vi "SPI Communication.vi"() -> ()   [LabVIEW 2023]
doc: "Overview\nDemonstrates how to use the NI-Digital Pattern Driver API to create and configure an instrument session and to burst a pattern on the digital pattern instrument using a start trigger."
uses:
  <instrlib>/niDigital/niDigital.llb/niDigital Pin State.ctl
  <instrlib>/niDigital/niDigital.llb/niDigital Data Mapping.ctl
  <instrlib>/niDigital/niDigital.llb/niDigital Bit Order.ctl
  <instrlib>/niDigital/niDigital.llb/niDigital Write Static Pin State.ctl
  <instrlib>/niDigital/niDigital.llb/niDigital Selected Function.ctl
  <instrlib>/niDigital/niDigital.llb/niDigital Load Specifications Levels and Timing (Single).vi
  <instrlib>/niDigital/niDigital.llb/niDigital Create Source Waveform (Serial).vi
  <instrlib>/niDigital/niDigital.llb/niDigital Create Capture Waveform (Serial).vi
  <instrlib>/niDigital/niDigital.llb/niDigital Write Source Waveform (Site Unique U32).vi
  <instrlib>/niDigital/niDigital.llb/niDigital Burst Pattern (Pass Fail).vi
  <instrlib>/niDigital/niDigital.llb/niDigital Output Function.ctl
panel:
  out "Command Value hex":u32[](array[numeric]) format="%.0x"
  in  "Write/Read":bool
  out "Command Value":u32[](array[numeric])
  out "Digital Data Out":bool[][](array[boolean])
  out "Burst Passed":bool
  out "DUT up":bool
  in  "LowStop":bool
  out "Read Value":u32[](array[numeric]) format="%.0x"
  in  "Write Value":u8[](array[numeric])=[16] format="%.0x"
  in  "Register Address":u8[](array[numeric])=[16] format="%.0x"
  in  "Digital Pattern Resource":refnum<k15>="HSD_6571_C02_S03" caption="resource name"
  in  "Debugg":bool
  in  "Write":bool
  in  "Read":bool
  out "Sequence Flags":bool[](array[boolean])
  out "Sequence Register":i32[](array[numeric])
  out "DIO State":cluster{"channel list":string, "data":T1}[](array[cluster]) {"data" items=["0"=0, "1"=1, "L"=3, "H"=4, "X"=5, "M"=6, "V"=7, "D"=8, "E"=9, "Not A Pin State"=254, "Pin State Not Acquired"=255]}
  out "error out":errorcluster
  # "!"
  # "In CTRL_REG1 set bit 1 to select 3 wire SPI instead of 4 wire.\nBei default it is 0."
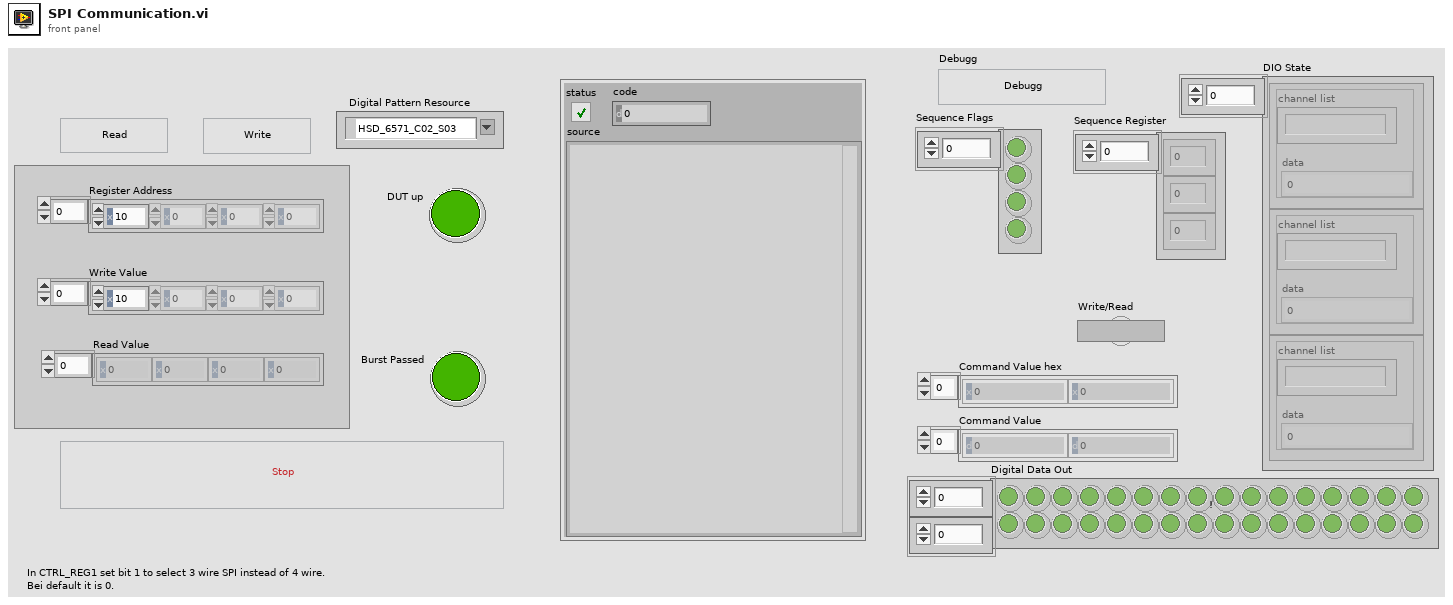
[diagram p1: front panel]
types:
  T1 = typedef "niDigital Pin State.ctl" = u8
  T2 = typedef "niDigital Bit Order.ctl" = i32
  T3 = typedef "niDigital Data Mapping.ctl" = i32
  T4 = typedef "niDigital Output Function.ctl" = i32
  T5 = typedef "niDigital Selected Function.ctl" = i32
  T6 = typedef "niDigital Write Static Pin State.ctl" = u8
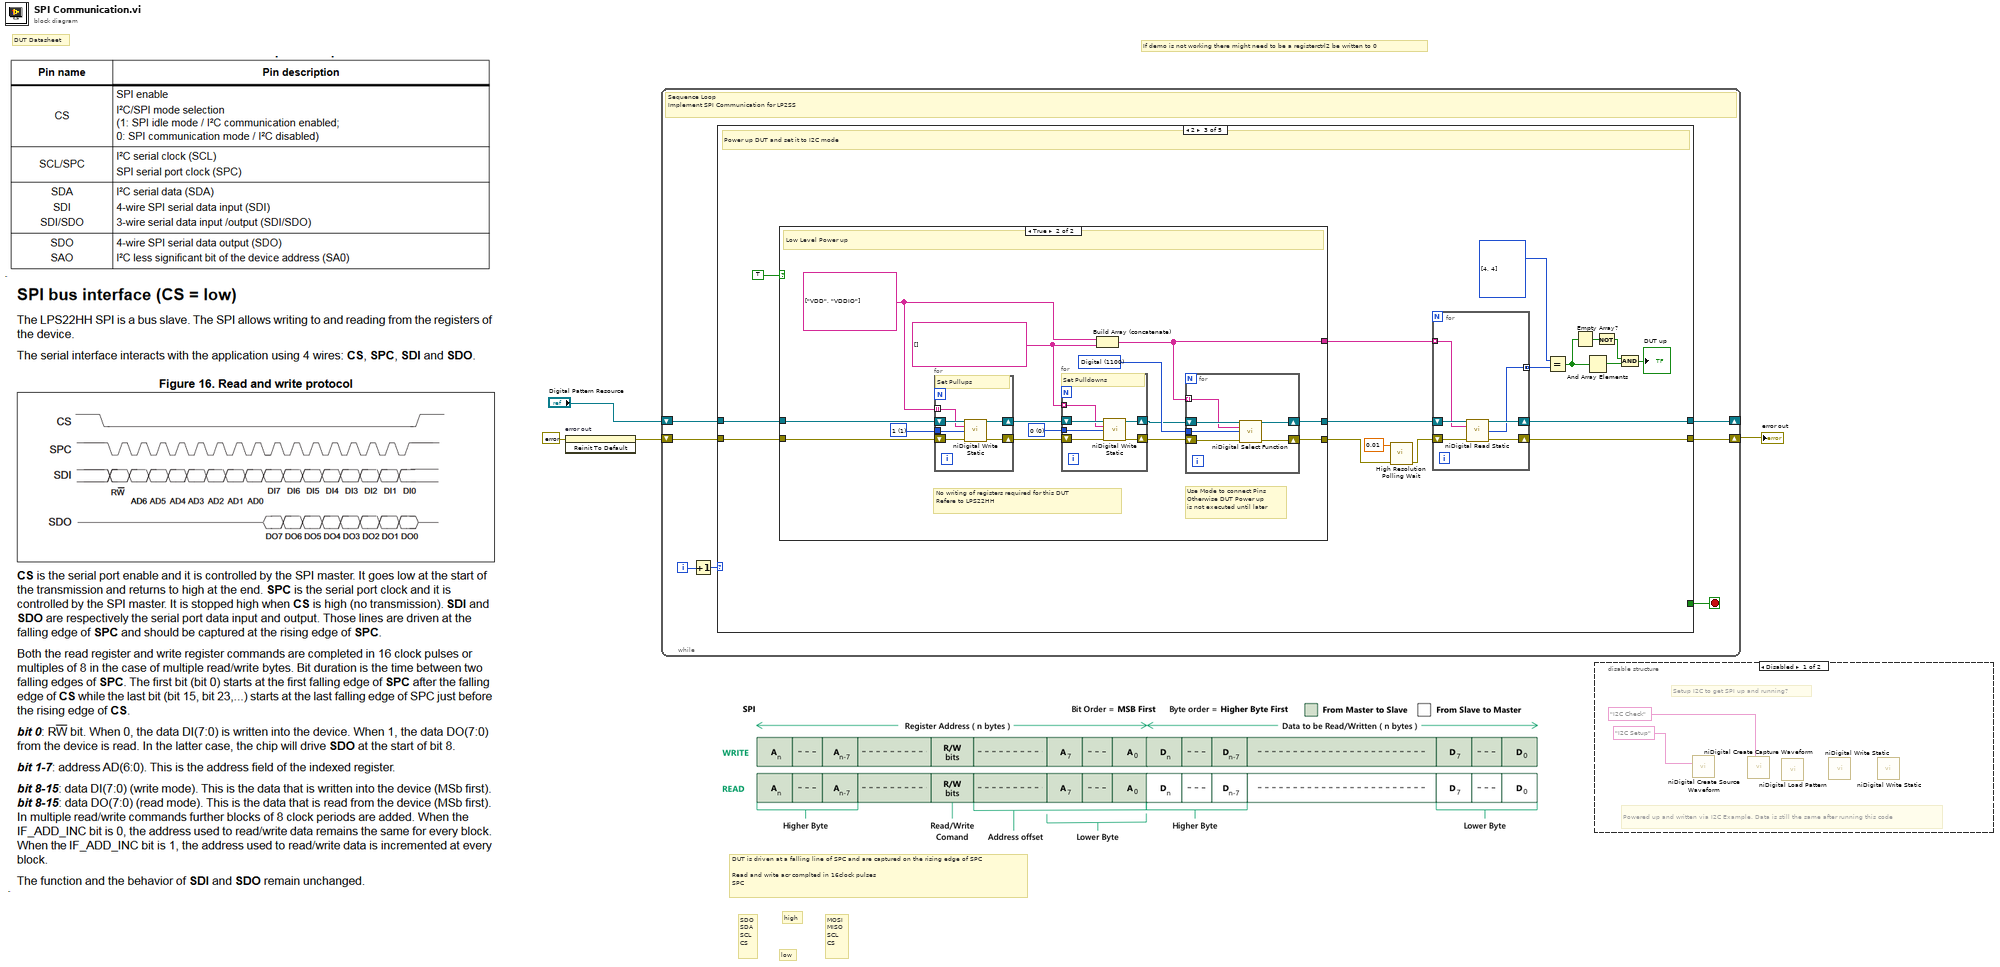
[diagram p0: block diagram]
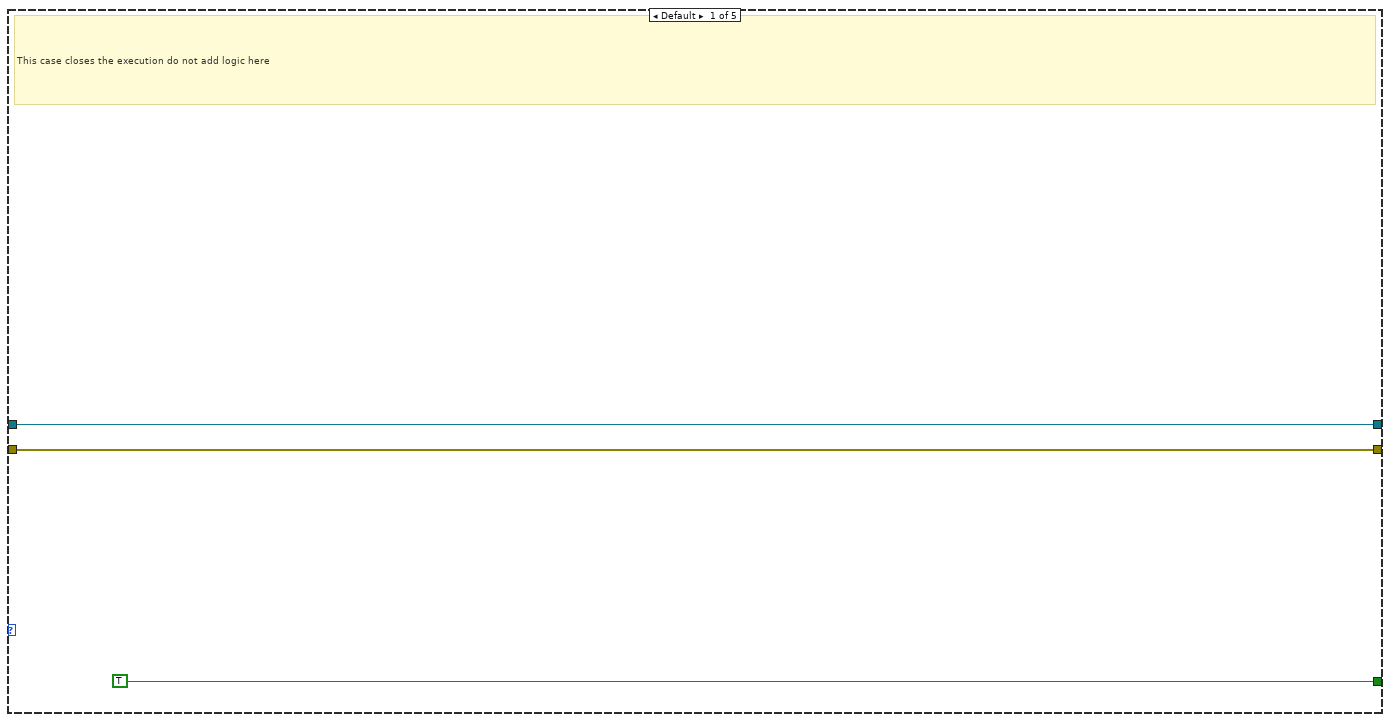
[diagram p3: hidden frame]
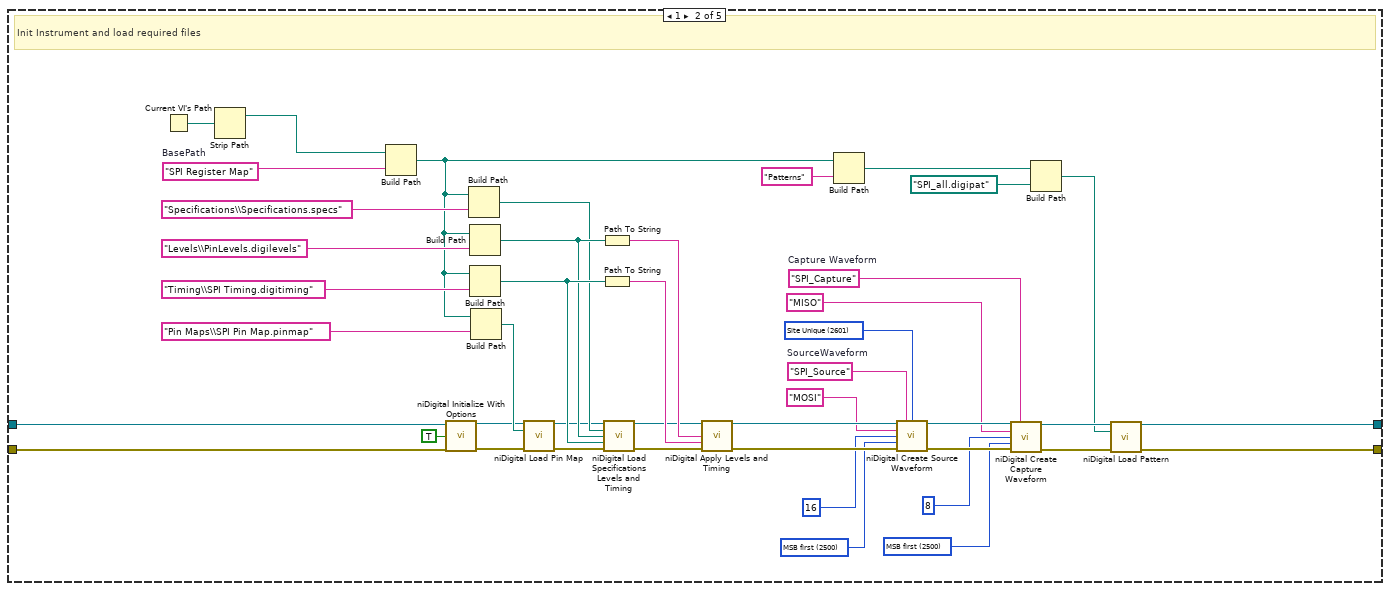
[diagram p4: hidden frame]
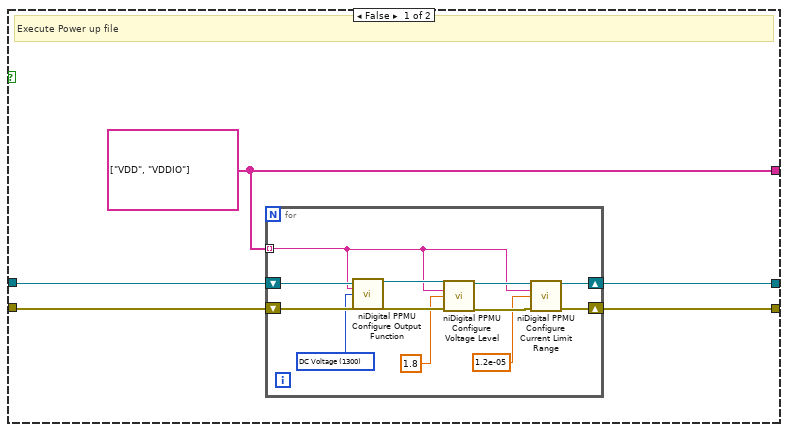
[diagram p5: hidden frame]
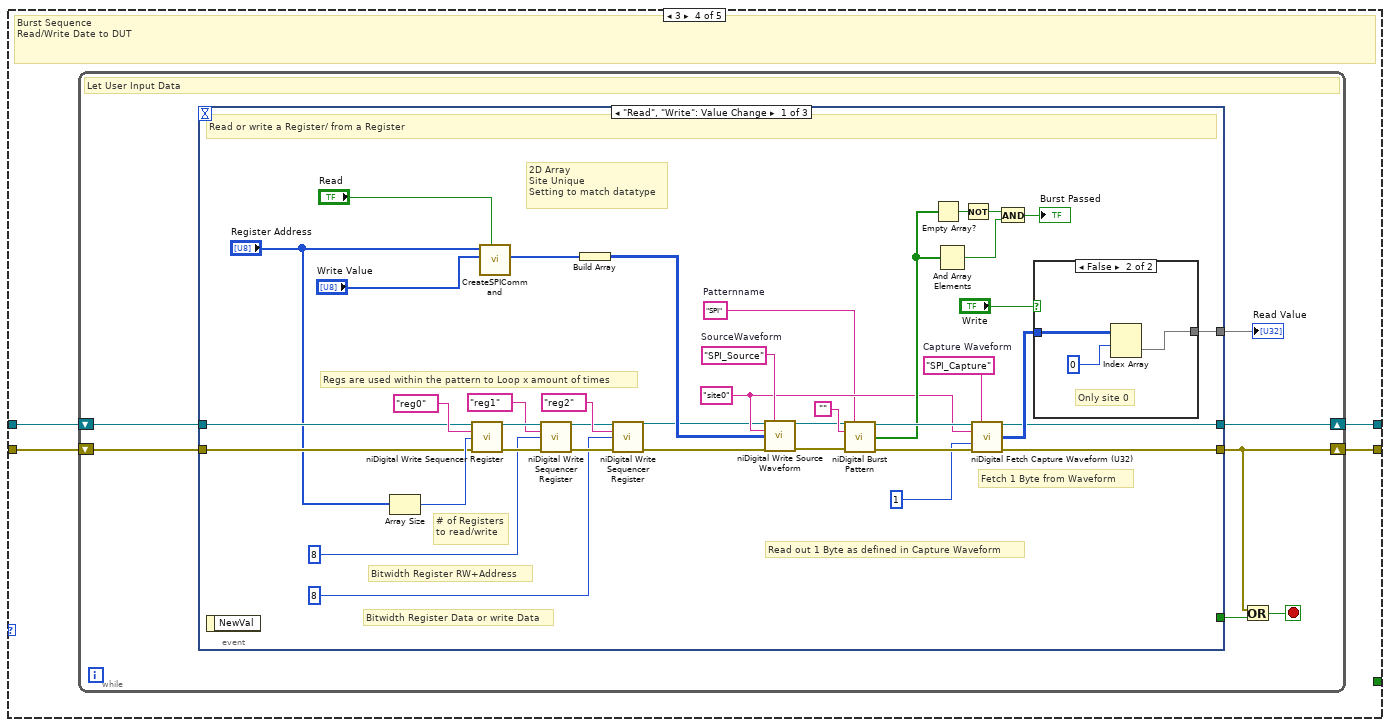
[diagram p6: hidden frame]
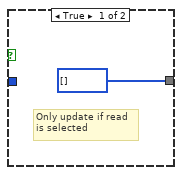
[diagram p7: hidden frame]
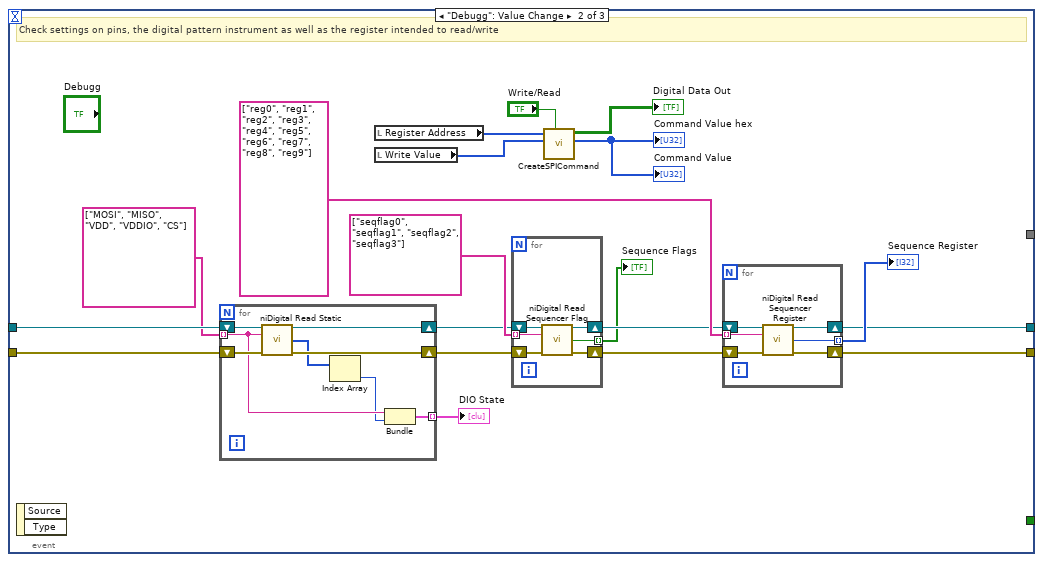
[diagram p8: hidden frame]
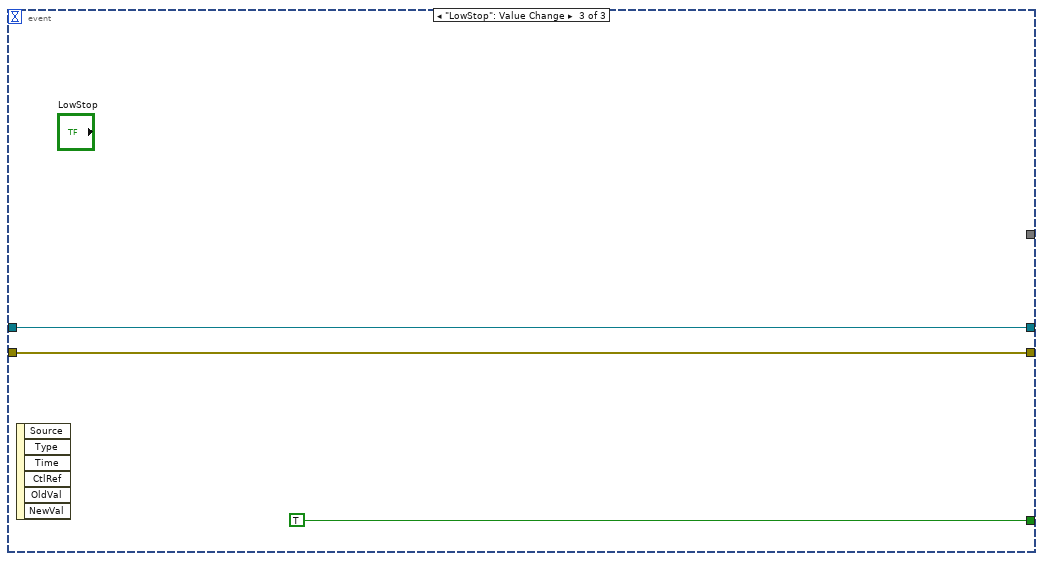
[diagram p9: hidden frame]
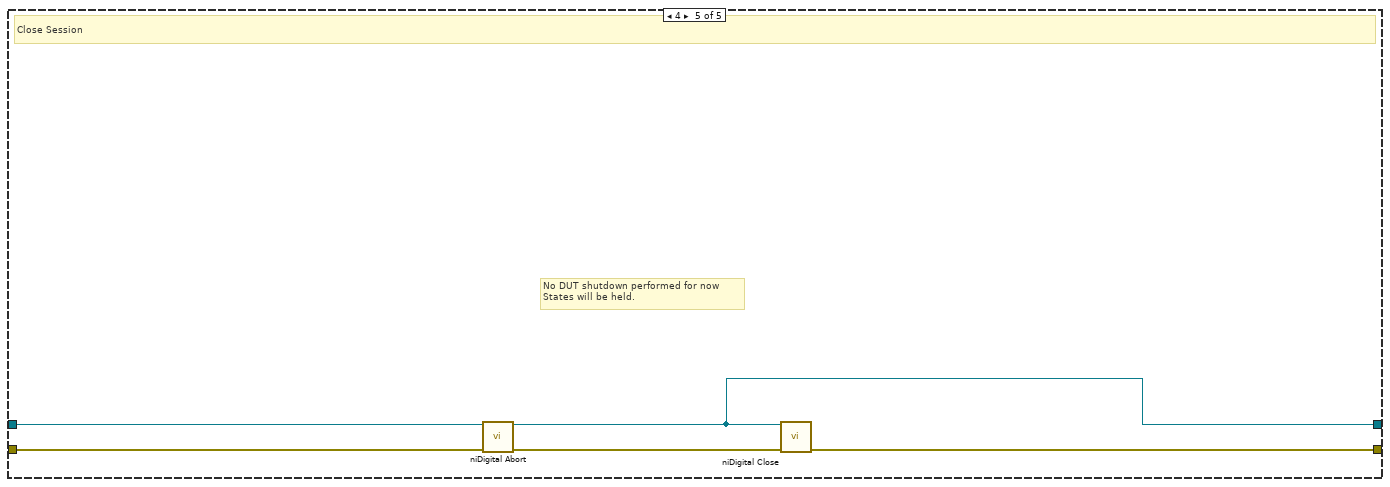
[diagram p10: hidden frame]
diagram:
  # "If demo is not working there might need to be a registerctrl2 be written to 0"
  # "MOSI\nMISO\nSCL\nCS"
  # "high"
  # "low"
  # "SDO\nSDA\nSCL\nCS"
  # "DUT Datasheet"
  # "DUT is driven at a falling line of SPC and are captured on the rising edge of SPC\n\nRead and write acr complted in 16clock pulses\nSPC"
  n1 = invoke on="error out" class="Clust (strict)" method="Reinit To Default"(error in=errorcluster {"status"=FALSE, "code"=0, "source"=""} ("error out")) -> (error out=w3:errorcluster)  [unwired: 2 in, 2 out]
  n2 = while {
    shift-right: [w11] -> w2
    shift-left: w3 -> [w7]
    shift-right: [w6] -> _
    shift-left: "Digital Pattern Resource" -> [w5]
    i -> [w9]
    stop <- w10 stop-if-true
    # "Sequence Loop\nImplement SPI Communication for LP2SS"
    n3 = Increment(x=w9) -> (x+1=w8:i32)
    n4 = case shown="2" w8 {
      tunnel: [w12 w37 w72 w134 w229] -> w6
      tunnel: w5 -> [w12 w28 w74 w133 w227]
      tunnel: w7 -> [w13 w27 w75 w132 w230]
      tunnel: [w13 w38 w73 w131 w231] -> w11
      tunnel: [TRUE _ _ _ _] -> w10
      frame Default {
        # "This case closes the execution do not add logic here"
      }
      frame 1 {
        w16 = T2 2500 items=["MSB first"=2500, "LSB first"=2501] ("bit order")
        w21 = T3 2601 items=["Broadcast"=2600, "Site Unique"=2601] ("data mapping")
        w22 = "SPI_Source"  # SourceWaveform
        w17 = T2 2500 items=["MSB first"=2500, "LSB first"=2501] ("bit order")
        w24 = "SPI_Capture"  # Capture Waveform
        w34 = "SPI Register Map"  # BasePath
        # "Init Instrument and load required files"
        n5 = Current VI's Path() -> (path=w33:path)
        n6 = Strip Path(path=w33) -> (stripped path=w32:path)  [unwired: 1 out]
        n7 = Build Path(base path=w32, name or relative path=w34) -> (appended path=w29:path)
        n8 = call <instrlib>:"niDigital Initialize With Options.vi"("resource name"=w28, "reset (T)"=TRUE, "error in"=w27) -> ("instrument handle"=w50:refnum<k15>, "error out"=w51:errorcluster)  [unwired: 11 in]
        n9 = Build Path(base path=w29, name or relative path="Specifications\\Specifications.specs") -> (appended path=w56:path)
        n10 = Build Path(base path=w29, name or relative path="Levels\\PinLevels.digilevels") -> (appended path=w57:path)
        n11 = Build Path(base path=w29, name or relative path="Timing\\SPI Timing.digitiming") -> (appended path=w58:path)
        n12 = Build Path(base path=w29, name or relative path="Pin Maps\\SPI Pin Map.pinmap") -> (appended path=w55:path)
        n13 = call <instrlib>:"niDigital Load Pin Map.vi"("instrument handle"=w50, "pin map file"=w55, "error in"=w51) -> ("instrument handle out"=w53:refnum<k15>, "error out"=w54:errorcluster)  [unwired: 11 in]
        n14 = Path To String(path=w57) -> (string=w52:string)
        n15 = Path To String(path=w58) -> (string=w49:string)
        n16 = call-poly <instrlib>:"niDigital Load Specifications Levels and Timing.vi"("instrument handle"=w53, "specifications file path"=w56, "levels file path"=w57, "timing file path"=w58, "error in"=w54) -> ("instrument handle out"=w45:refnum<k15>, "error out"=w46:errorcluster)  [unwired: 9 in]
        n17 = call <instrlib>:"niDigital Apply Levels and Timing.vi"("instrument handle"=w45, "levels sheet"=w52, "timing sheet"=w49, "error in"=w46) -> ("instrument handle out"=w48:refnum<k15>, "error out"=w47:errorcluster)  [unwired: 10 in]
        n18 = Build Path(base path=w29, name or relative path="Patterns") -> (appended path=w30:path)
        n19 = call-poly <instrlib>:"niDigital Create Source Waveform.vi"("instrument handle"=w48, "waveform name"=w22, "data mapping"=w21, "pin list"="MOSI", "sample width"=u32 16, "bit order"=w17, "error in"=w47) -> ("instrument handle out"=w25:refnum<k15>, "error out"=w26:errorcluster)  [unwired: 7 in]
        n20 = call-poly <instrlib>:"niDigital Create Capture Waveform.vi"("instrument handle"=w25, "waveform name"=w24, "pin list"="MISO", "sample width"=u32 8, "bit order"=w16, "error in"=w26) -> ("instrument handle out"=w40:refnum<k15>, "error out"=w39:errorcluster)  [unwired: 8 in]
        n21 = Build Path(base path=w30, name or relative path=path "SPI_all.digipat" ("pattern file")) -> (appended path=w35:path)
        n22 = call <instrlib>:"niDigital Load Pattern.vi"("instrument handle"=w40, "pattern file"=w35, "error in"=w39) -> ("instrument handle out"=w37:refnum<k15>, "error out"=w38:errorcluster)  [unwired: 11 in]
      }
      frame 2 {
        w63 = T1[] [4, 4] items=["0"=0, "1"=1, "L"=3, "H"=4, "X"=5, "M"=6, "V"=7, "D"=8, "E"=9, "Not A Pin State"=254, "Pin State Not Acquired"=255]
        # "Power up DUT and set it to I2C mode"
        n23 = case shown="True" TRUE {
          tunnel: w75 -> [w79 w106]
          tunnel: w74 -> [w80 w105]
          tunnel: [w77 w99] -> w65
          tunnel: [w78 w98] -> w61
          tunnel: [w76 w96] -> w64
          frame False {
            w76 = string[] ["VDD", "VDDIO"] ("channel list")
            # "Execute Power up file"
            n24 = for {
              shift-right: [w84] -> w77
              shift-left: w80 -> [w92]
              shift-right: [w85] -> w78
              shift-left: w79 -> [w91]
              tunnel: w76 -> [w82] mode=indexing
              w88 = T4 1300 items=["DC Voltage"=1300, "DC Current"=1301] ("output function")
              n25 = call <instrlib>:"niDigital PPMU Configure Output Function.vi"("instrument handle"=w92, "channel list"=w82, "output function"=w88, "error in"=w91) -> ("instrument handle out"=w90:refnum<k15>, "error out"=w89:errorcluster)  [unwired: 10 in]
              n26 = call <instrlib>:"niDigital PPMU Configure Voltage Level.vi"("instrument handle"=w90, "channel list"=w82, "voltage level (V)"=1.8, "error in"=w89) -> ("instrument handle out"=w83:refnum<k15>, "error out"=w86:errorcluster)  [unwired: 10 in]
              n27 = call <instrlib>:"niDigital PPMU Configure Current Limit Range.vi"("instrument handle"=w83, "channel list"=w82, "current limit range (A)"=1.2e-05 ("current limit (A)"), "error in"=w86) -> ("instrument handle out"=w84:refnum<k15>, "error out"=w85:errorcluster)  [unwired: 10 in]
            }
          }
          frame True {
            w97 = T5 1100 items=["Digital"=1100, "PPMU"=1101, "Off"=1102, "Disconnect"=1103, "RIO"=1104] ("function")
            w100 = string[] [] ("channel list")
            w103 = T6 0 items=["0"=0, "1"=1, "X"=5] ("state")
            w94 = string[] ["VDD", "VDDIO"] ("channel list")
            w104 = T6 1 items=["0"=0, "1"=1, "X"=5] ("state")
            # "Use Mode to connect Pins\nOtherwise DUT Power up \nis not executed until later"
            # "No writing of registers required for this DUT\nRefere to LPS22HH"
            # "Low Level Power up"
            n28 = for {
              tunnel: w104 -> [w122]
              tunnel: w94 -> [w121] mode=indexing
              shift-right: [w120] -> w102
              shift-left: w105 -> [w123]
              shift-right: [w119] -> w101
              shift-left: w106 -> [w124]
              # "Set Pullups"
              n29 = call <instrlib>:"niDigital Write Static.vi"("instrument handle"=w123, "channel list"=w121, "state"=w122, "error in"=w124) -> ("instrument handle out"=w120:refnum<k15>, "error out"=w119:errorcluster)  [unwired: 10 in]
            }
            n30 = for {
              tunnel: w103 -> [w116]
              tunnel: w100 -> [w115] mode=indexing
              shift-right: [w114] -> w95
              shift-left: w101 -> [w118]
              shift-right: [w113] -> w93
              shift-left: w102 -> [w117]
              # "Set Pulldowns"
              n31 = call <instrlib>:"niDigital Write Static.vi"("instrument handle"=w117, "channel list"=w115, "state"=w116, "error in"=w118) -> ("instrument handle out"=w113:refnum<k15>, "error out"=w114:errorcluster)  [unwired: 10 in]
            }
            n32 = Build Array (concatenate)(w94, w100) -> (w96:string[])
            n33 = for {
              shift-right: [w111] -> w99
              shift-left: w93 -> [w110]
              shift-right: [w112] -> w98
              shift-left: w95 -> [w109]
              tunnel: w97 -> [w108]
              tunnel: w96 -> [w107] mode=indexing
              n34 = call <instrlib>:"niDigital Select Function.vi"("instrument handle"=w110, "channel list"=w107, "function"=w108, "error in"=w109) -> ("instrument handle out"=w111:refnum<k15>, "error out"=w112:errorcluster)  [unwired: 10 in]
            }
          }
        }
        n35 = call <vilib>:"High Resolution Polling Wait.vi"("error in (no error)"=w61, "seconds to wait"=0.01) -> ("error out"=w60:errorcluster)  [unwired: 9 in]
        n36 = for {
          shift-right: [w129] -> w73
          shift-left: w60 -> [w130]
          shift-right: [w127] -> w72
          shift-left: w65 -> [w128]
          tunnel: w64 -> [w126] mode=indexing
          tunnel: [w125] -> w71 mode=concatenating
          n37 = call <instrlib>:"niDigital Read Static.vi"("instrument handle"=w128, "channel list"=w126, "error in"=w130) -> ("instrument handle out"=w127:refnum<k15>, "data"=w125:T1[], "error out"=w129:errorcluster)  [unwired: 10 in]
        }
        n38 = Equal?(x=w63, y=w71) -> (x = y?=w68:bool[])
        n39 = Empty Array?(array=w68) -> (empty?=w70:bool)
        n40 = And Array Elements(Boolean array=w68) -> (logical AND=w67:bool)
        n41 = Not(x=w70) -> (.not. x?=w69:bool)
        n42 = And(x=w69, y=w67) -> (x .and. y?=→"DUT up":bool)
      }
      frame 3 {
        # "Burst Sequence\nRead/Write Date to DUT"
        n43 = while {
          shift-right: [w135] -> w131
          shift-left: w132 -> [w136]
          shift-right: [w140] -> w134
          shift-left: w133 -> [w141]
          stop <- w138 stop-if-true
          # "Let User Input Data"
          n44 = event shown="[0] \"Read\", \"Write\": Value Change" {
            selector: _ -> [_ _ _]
            dyn-events: _ -> [_ _ _]
            timeout: _ -> [_ _ _]
            tunnel: w136 -> [w149 w199 w226]
            tunnel: w141 -> [w148 w196 w225]
            tunnel: [w175 w191 w226] -> w135
            tunnel: [w174 w187 w225] -> w140
            tunnel: [_ _ TRUE ("stop")] -> w139
            tunnel: [w179 _ _] -> w137
            event "Read", "Write": Value Change {
              w147 = "SPI"  # Patternname
              w155 = "SPI_Capture"  # Capture Waveform
              w156 = "SPI_Source"  # SourceWaveform
              w154 = "site0" ("site list")
              # "Read out 1 Byte as defined in Capture Waveform"
              # "Bitwidth Register Data or write Data"
              # "Regs are used within the pattern to Loop x amount of times"
              # "2D Array \nSite Unique \nSetting to match datatype"
              # "Bitwidth Register RW+Address"
              # "# of Registers\nto read/write"
              # "Fetch 1 Byte from Waveform"
              # "Read or write a Register/ from a Register"
              n45 = event-data() -> ()  [unwired: 1 in, 1 out]
              n46 = Array Size(array="Register Address") -> (size(s)=w157:i32)
              n47 = call <instrlib>:"niDigital Write Sequencer Register.vi"("instrument handle"=w148, "sequencer register"="reg0", "value"=w157, "error in"=w149) -> ("instrument handle out"=w163:refnum<k15>, "error out"=w162:errorcluster)  [unwired: 10 in]
              n48 = call "CreateSPICommand.vi"("Write/Read"="Read", "Write Value"="Write Value", "Register Address"="Register Address") -> ("Command Value"=w142:u32[])  [unwired: 7 in, 1 out]
              n49 = call <instrlib>:"niDigital Write Sequencer Register.vi"("instrument handle"=w163, "sequencer register"="reg1", "value"=8, "error in"=w162) -> ("instrument handle out"=w160:refnum<k15>, "error out"=w161:errorcluster)  [unwired: 10 in]
              n50 = Build Array(w142) -> (w158:u32[][])
              n51 = call <instrlib>:"niDigital Write Sequencer Register.vi"("instrument handle"=w160, "sequencer register"="reg2", "value"=8, "error in"=w161) -> ("instrument handle out"=w153:refnum<k15>, "error out"=w152:errorcluster)  [unwired: 10 in]
              n52 = call-poly <instrlib>:"niDigital Write Source Waveform.vi"("instrument handle"=w153, "waveform name"=w156, "site list"=w154, "waveform data"=w158, "error in"=w152) -> ("instrument handle out"=w172:refnum<k15>, "error out"=w171:errorcluster)  [unwired: 9 in]
              n53 = call-poly <instrlib>:"niDigital Burst Pattern.vi"("instrument handle"=w172, "start label"=w147, "site list"="", "error in"=w171) -> ("instrument handle out"=w176:refnum<k15>, "pass"=w169:bool[], "error out"=w177:errorcluster)  [unwired: 9 in]
              n54 = Empty Array?(array=w169) -> (empty?=w170:bool)
              n55 = And Array Elements(Boolean array=w169) -> (logical AND=w167:bool)
              n56 = Not(x=w170) -> (.not. x?=w168:bool)
              n57 = call <instrlib>:"niDigital Fetch Capture Waveform (U32).vi"("instrument handle"=w176, "waveform name"=w155, "site list"=w154, "samples to read"=1, "error in"=w177) -> ("instrument handle out"=w174:refnum<k15>, "data"=w180:u32[][], "error out"=w175:errorcluster)  [unwired: 8 in]
              n58 = And(x=w168, y=w167) -> (x .and. y?=→"Burst Passed":bool)
              n59 = case shown="False" "Write" {
                tunnel: w180 -> [_ w182]
                tunnel: [u32[] [] ("data") w184] -> w179
                frame True {
                  # "Only update if read\nis selected"
                }
                frame False {
                  # "Only site 0"
                  n60 = Index Array(array=w182, index (row)=0) -> (element=w184:u32[])  [unwired: 1 in]
                }
              }
            }
            event "Debugg": Value Change {
              # "Check settings on pins, the digital pattern instrument as well as the register intended to read/write"
              n61 = event-data() -> ()  [unwired: 1 in, 2 out]
              n62 = for {
                tunnel: string[] ["MOSI", "MISO", "VDD", "VDDIO", "CS"] ("channel list") -> [w207] mode=indexing
                shift-right: [w210] -> w198
                shift-left: w199 -> [w211]
                shift-right: [w209] -> w197
                shift-left: w196 -> [w208]
                tunnel: [w206] -> w194 mode=indexing
                n63 = call <instrlib>:"niDigital Read Static.vi"("instrument handle"=w208, "channel list"=w207, "error in"=w211) -> ("instrument handle out"=w209:refnum<k15>, "data"=w205:T1[], "error out"=w210:errorcluster)  [unwired: 10 in]
                n64 = Index Array(array=w205) -> (element=w204:T1)  [unwired: 1 in]
                n65 = Bundle("channel list"=w207, "state"=w204) -> (w206:cluster{"channel list":string, "state":T1})  [unwired: 1 in]
              }
              "DIO State" <- w194
              n66 = local read "Register Address"() -> (w190:u8[])
              n67 = local read "Write Value"() -> (w189:u8[])
              n68 = for {
                tunnel: string[] ["seqflag0", "seqflag1", "seqflag2", "seqflag3"] ("sequencer flag") -> [w216] mode=indexing
                tunnel: [w215] -> w193 mode=indexing
                shift-right: [w214] -> w201
                shift-left: w198 -> [w217]
                shift-right: [w213] -> w200
                shift-left: w197 -> [w212]
                n69 = call <instrlib>:"niDigital Read Sequencer Flag.vi"("instrument handle"=w212, "sequencer flag"=w216, "error in"=w217) -> ("instrument handle out"=w213:refnum<k15>, "state"=w215:bool, "error out"=w214:errorcluster)  [unwired: 10 in]
              }
              "Sequence Flags" <- w193
              n70 = call "CreateSPICommand.vi"("Write/Read"="Write/Read", "Write Value"=w189, "Register Address"=w190) -> ("Command Value"=→"Command Value" →"Command Value hex":u32[], "Command Bitstream"=→"Digital Data Out":bool[][])  [unwired: 7 in]
              n71 = for {
                tunnel: string[] ["reg0", "reg1", "reg2", "reg3", "reg4", "reg5", "reg6", "reg7", "reg8", "reg9"] ("sequencer register") -> [w221] mode=indexing
                tunnel: [w220] -> w192 mode=indexing
                shift-right: [w222] -> w191
                shift-left: w201 -> [w219]
                shift-right: [w223] -> w187
                shift-left: w200 -> [w218]
                n72 = call <instrlib>:"niDigital Read Sequencer Register.vi"("instrument handle"=w218, "sequencer register"=w221, "error in"=w219) -> ("instrument handle out"=w223:refnum<k15>, "value"=w220:i32, "error out"=w222:errorcluster)  [unwired: 10 in]
              }
              "Sequence Register" <- w192
            }
            event "LowStop": Value Change {
              n73 = event-data() -> ()  [unwired: 1 in, 6 out]
            }
          }
          "Read Value" <- w137
          n74 = Or(x=w135, y=w139) -> (x .or. y?=w138:bool)
        }
      }
      frame 4 {
        # "No DUT shutdown performed for now\nStates will be held."
        # "Close Session"
        n75 = call <instrlib>:"niDigital Abort.vi"("instrument handle"=w227, "error in"=w230) -> ("instrument handle out"=w229:refnum<k15>, "error out"=w228:errorcluster)  [unwired: 12 in]
        n76 = call <instrlib>:"niDigital Close.vi"("instrument handle"=w229, "error in"=w228) -> ("error out"=w231:errorcluster)  [unwired: 13 in]
      }
    }
  }
  "error out" <- w2
  n77 = disable-structure shown="Disabled" {
    frame Disabled {
      # "Powered up and written via I2C Example. Data is still the same after running this code"
      # "Setup I2C to get SPI up and running?"
      n78 = call-poly <instrlib>:"niDigital Create Source Waveform.vi"("pin list"="I2C Setup") -> ()  [unwired: 13 in, 2 out]
      n79 = call-poly <instrlib>:"niDigital Create Capture Waveform.vi"("waveform name"="I2C Check" ("pin list")) -> ()  [unwired: 13 in, 2 out]
      n80 = call <instrlib>:"niDigital Load Pattern.vi"() -> ()  [unwired: 14 in, 2 out]
      n81 = call <instrlib>:"niDigital Write Static.vi"() -> ()  [unwired: 14 in, 2 out]
      n82 = call <instrlib>:"niDigital Write Static.vi"() -> ()  [unwired: 14 in, 2 out]
    }
    frame Enabled {
    }
  }
